vi "UDP - Get IP Addresses.vi"(8 "error in":errorcluster, 11 "IP Address":string[](array[string])) -> (0 "error out":errorcluster, 3 "IP Addresses":string[](array[string]))   [LabVIEW 2019]
uses:
  Controls/Global - Data UDP.vi
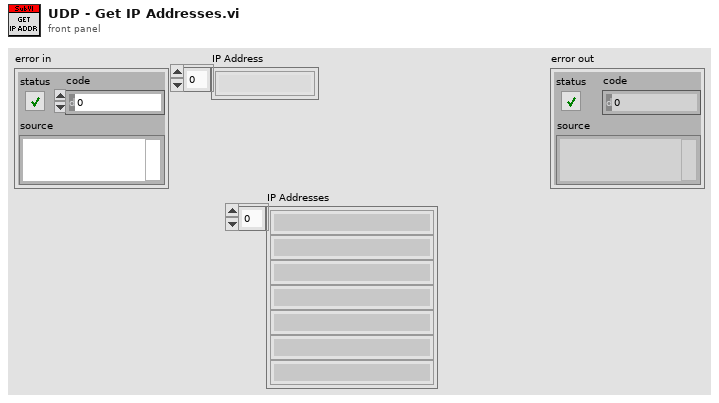
[diagram p1: front panel]
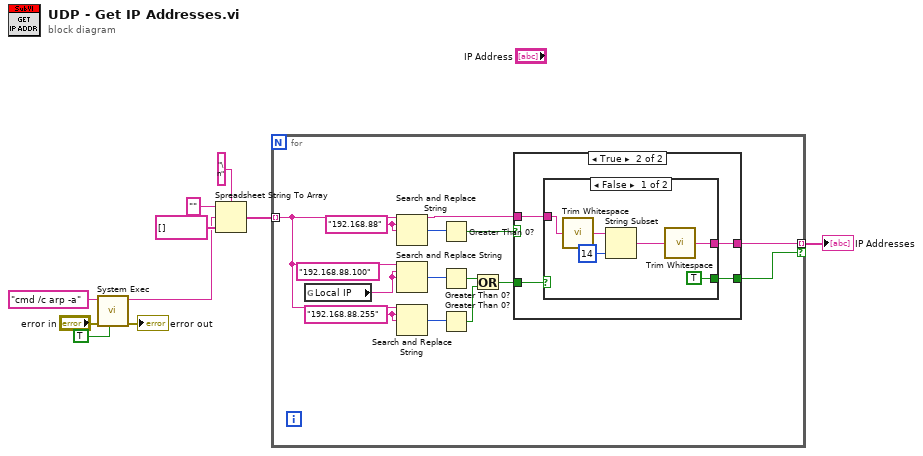
[diagram p0: block diagram]
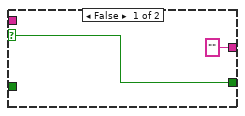
[diagram p2: hidden frame]
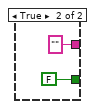
[diagram p3: hidden frame]
diagram:
  n1 = call <vilib>:"System Exec.vi"("run minimized? (F)"=TRUE, "error in (no error)"="error in", "command line"="cmd /c arp -a") -> ("error out"=→"error out":errorcluster, "standard output"=w6:string)  [unwired: 5 in, 2 out]
  n2 = Spreadsheet String To Array(delimiter (Tab)="\n", format string="", spreadsheet string=w6, array type (2D Dbl)=string[] []) -> (array=w4:string[])
  n3 = for {
    tunnel: w4 -> [w15] mode=indexing
    tunnel: [w19] -> w3 mode=indexing if=w18
    w17 = "192.168.88.255" ("search string")
    (unwired) "192.168.88.100" ("search string")
    w24 = "192.168.88" ("search string")
    n4 = global read "Global - Data UDP.vi" "Local IP"() -> (w11:string)
    n5 = Search and Replace String(input string=w15, search string=w24, replace string=w24) -> (result string=w20:string, number of replacements=w23:i32)  [unwired: 5 in, 2 out]
    n6 = Search and Replace String(input string=w15, search string=w11, replace string=w11) -> (number of replacements=w22:i32)  [unwired: 5 in, 3 out]
    n7 = Search and Replace String(input string=w15, search string=w17, replace string=w17) -> (number of replacements=w16:i32)  [unwired: 5 in, 3 out]
    n8 = Greater Than 0?(x=w23) -> (x > 0?=w21:bool)
    n9 = Greater Than 0?(x=w22) -> (x > 0?=w14:bool)
    n10 = Greater Than 0?(x=w16) -> (x > 0?=w13:bool)
    n11 = Or(x=w14, y=w13) -> (x .or. y?=w12:bool)
    n12 = case shown="True" w21 {
      selector: w21 -> [w25 _]
      tunnel: w20 -> [_ w30]
      tunnel: ["" ("trimmed string") w29] -> w19
      tunnel: [w25 w27] -> w18
      tunnel: w12 -> [_ w28]
      frame False {
      }
      frame True {
        n13 = case shown="False" w28 {
          tunnel: w30 -> [w33 _]
          tunnel: [w32 "" ("trimmed string")] -> w29
          tunnel: [TRUE FALSE] -> w27
          frame False {
            n14 = call <vilib>:"Trim Whitespace.vi"("string"=w33) -> ("trimmed string"=w34:string)  [unwired: 1 in]
            n15 = String Subset(string=w34, length (rest)=14 ("length (rest)")) -> (substring=w36:string)  [unwired: 1 in]
            n16 = call <vilib>:"Trim Whitespace.vi"("string"=w36) -> ("trimmed string"=w32:string)  [unwired: 1 in]
          }
          frame True {
          }
        }
      }
    }
  }
  "IP Addresses" <- w3
